vi "Add_File_Extension.vi"(10 "Extension":string, 11 "File Path In":path) -> (3 "File Path Out":path)   [LabVIEW 2012]
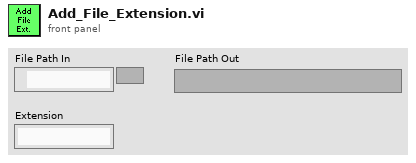
[diagram p1: front panel]
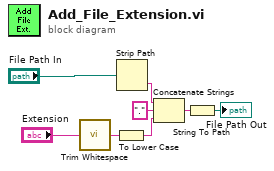
[diagram p0: block diagram]
diagram:
  n1 = call <vilib>:"Trim Whitespace.vi"("string"="Extension") -> ("trimmed string"=w2:string)  [unwired: 1 in]
  n2 = To Lower Case(string=w2) -> (all lower case string=w6:string)
  n3 = Strip Path(path="File Path In") -> (name=w4:string)  [unwired: 1 out]
  n4 = Concatenate Strings(w4, "." ("string"), w6) -> (w7:string)
  n5 = String To Path(string=w7) -> (path=→"File Path Out":path)
